vi "PreObjectInitialize.vi"(8 "error in (no error)":errorcluster, 11 "AFM.Asylum in":refnum<class "AFM_Driver.lvclass">) -> (0 "error out":errorcluster, 3 "AFM.Asylum out":refnum<class "AFM_Driver.lvclass">)   [LabVIEW 2019, in "AFM_Driver.lvclass"]
uses:
  AFM_Driver.lvclass
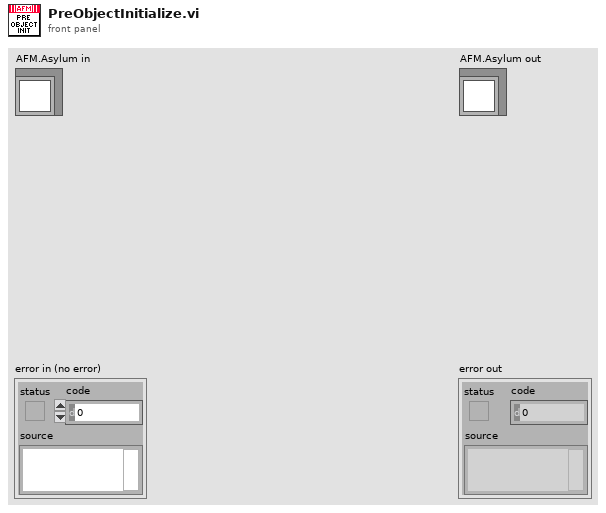
[diagram p1: front panel]
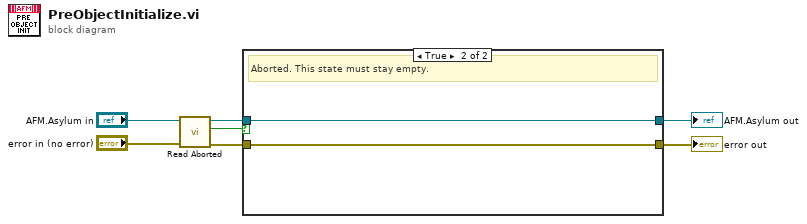
[diagram p0: block diagram]
diagram:
  n1 = call "Read Aborted.vi"("error in (no error)"="error in (no error)", "AFM_Driver in"="AFM.Asylum in") -> ("error out"=w1:errorcluster, "Aborted?"=w5:bool, "AFM_Driver out"=w4:refnum<class "AFM_Driver.lvclass">)  [unwired: 7 in]
  n2 = case shown="True" w5 {
    tunnel: w4 -> [w8 w11]
    tunnel: [w8 w11] -> w3
    tunnel: [w9 w10] -> w2
    tunnel: w1 -> [w9 w10]
    frame False {
      # "Not Aborted."
    }
    frame True {
      # "Aborted. This state must stay empty."
    }
  }
  "error out" <- w2
  "AFM.Asylum out" <- w3
